vi "To String.vi"(8 "error in (no error)":errorcluster, 11 "Double Float in":refnum<class "Abs_I16 Integer.lvclass">) -> (0 "error out":errorcluster, 2 "String":string, 3 "Double Float out":refnum<class "Abs_I16 Integer.lvclass">)   [LabVIEW 2021, in "Abs_I16 Integer.lvclass"]
uses:
  Abs_I16 Integer.lvclass
  C:/Program Files (x86)/National Instruments/LabVIEW 2021/vi.lib/TSA/Abstract Data Classes/Abs_Types/Numeric/Abs_Numeric.lvclass
  Numeric/Abs_Numeric.lvclass/Abs_Numeric.ctl
  Numeric/Properties/Read Units.vi
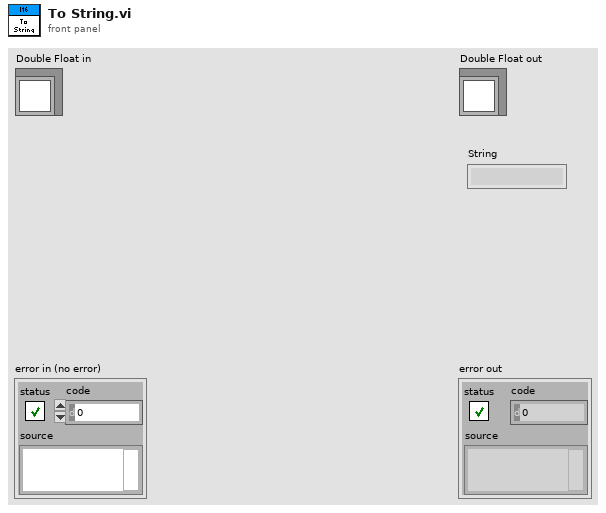
[diagram p1: front panel]
types:
  T1 = typedef "Abs_I16 Integer.lvclass/Type.ctl" = i16
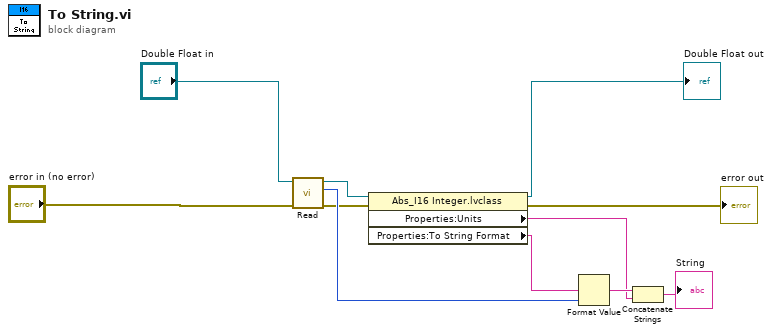
[diagram p0: block diagram]
diagram:
  n1 = call-dynamic "Read.vi"("error in (no error)"="error in (no error)", "Double Float.lvclass_340760 in"="Double Float in") -> ("error out"=w4:errorcluster, "Value"=w5:T1, "Double Float.lvclass_340760 out"=w6:refnum<class "Abs_I16 Integer.lvclass">)  [unwired: 7 in]
  n2 = property class="Abs_I16 Integer.lvclass"(reference=w6, error in=w4) -> (reference out=→"Double Float out":refnum<class "Abs_I16 Integer.lvclass">, error out=→"error out":errorcluster, "Properties:Units"=w1:string, "Properties:To String Format"=w7:string)
  n3 = Format Value(format string=w7, value (0)=w5) -> (output string=w3:string)  [unwired: 1 in]
  n4 = Concatenate Strings(w3, w1) -> (→"String":string)
